vi "Coarse and Fine Log Sweep.vi"(0 "Coarse Sweep":T1 {"End" format="%#_13g"; "Start" format="%#_13g"}, 5 "Fine Sweep":T1 {"End" format="%#_13g"; "Start" format="%#_13g"}, 11 "error in (no error)":errorcluster) -> (4 "Sweep Values":dbl[](array[numeric]), 15 "error out":errorcluster)   [LabVIEW 2020]
doc: "Coarse and Fine Log Sweep does a Logarthmic sweep for both input coarse and fine sweep parameters and combines the obtained sweep values to a single output array."
uses:
  Sweep Parameters.ctl
  <vilib>/Analysis/1siggen.llb/Ramp Pattern.vi
  <vilib>/Analysis/1siggen.llb/Ramp Pattern by Samples.vi
  <vilib>/Utility/error.llb/Error Cluster From Error Code.vi
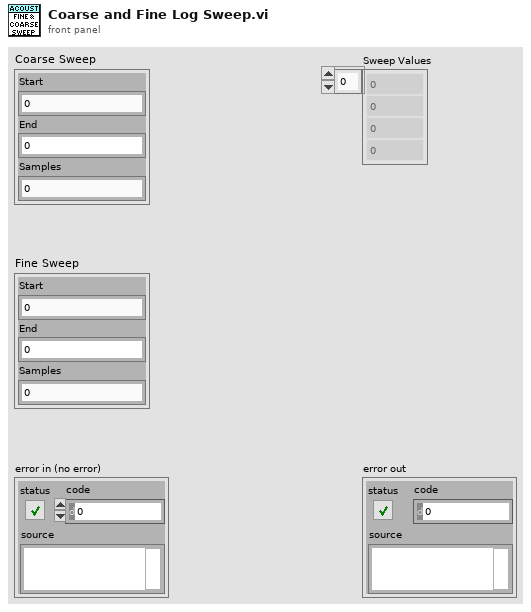
[diagram p1: front panel]
types:
  T1 = typedef "Sweep Parameters.ctl" = cluster{"Start":dbl, "End":dbl, "Samples":i32}
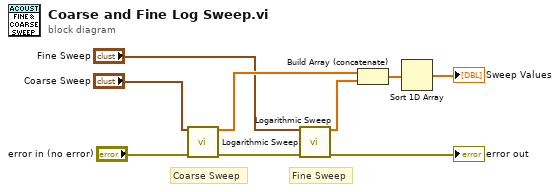
[diagram p0: block diagram]
diagram:
  # "Fine Sweep"
  # "Coarse Sweep"
  n1 = call "Logarithmic Sweep.vi"("Sweep Parameters"="Coarse Sweep", "error in (no error)"="error in (no error)") -> ("Ramp Pattern"=w7:dbl[], "error out"=w5:errorcluster)  [unwired: 12 in]
  n2 = call "Logarithmic Sweep.vi"("Sweep Parameters"="Fine Sweep", "error in (no error)"=w5) -> ("Ramp Pattern"=w6:dbl[], "error out"=→"error out":errorcluster)  [unwired: 12 in]
  n3 = Build Array (concatenate)(w7, w6) -> (w9:dbl[])
  n4 = Sort 1D Array(array=w9) -> (sorted array=→"Sweep Values":dbl[])
